vi "Write Y_index.vi"(4 "Find all":bool=TRUE, 6 "Parameter":string="_YQ01", 9 "Heater":string, 10 "EnumsAO":string[](array[string]), 11 "Heater in":refnum<class "Heater.lvclass">) -> (2 "Find":bool, 3 "Heater out":refnum<class "Heater.lvclass">)   [LabVIEW 2019, in "Heating.lvlib" / "Heater.lvclass"]
uses:
  Heater.lvclass
  Heater.lvclass/Heater.ctl
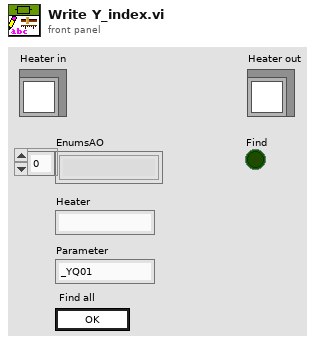
[diagram p1: front panel]
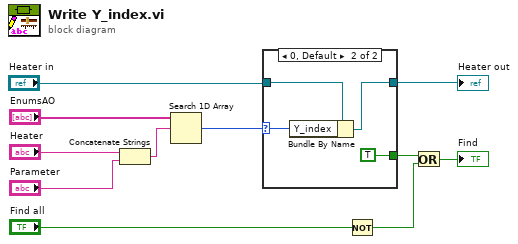
[diagram p0: block diagram]
diagram:
  n1 = Concatenate Strings("Heater", "Parameter") -> (w10:string)
  n2 = Search 1D Array(1D array="EnumsAO", element=w10) -> (index of element=w7:i32)  [unwired: 1 in]
  n3 = case shown="0, Default" w7 {
    selector: w7 -> [_ w14]
    tunnel: "Heater in" -> [w12 w16]
    tunnel: [w12 w15] -> w4
    tunnel: [_ TRUE] -> w6
    frame -1 {
    }
    frame 0, Default {
      n4 = Bundle By Name(cluster=w16, "Y_index"=w14) -> (w15:refnum<class "Heater.lvclass">)
    }
  }
  "Heater out" <- w4
  n5 = Not(x="Find all") -> (.not. x?=w1:bool)
  n6 = Or(x=w6, y=w1) -> (x .or. y?=→"Find":bool)
